vi "L42.vi"() -> ()   [LabVIEW 2014]
panel:
  in  "L42":dbl
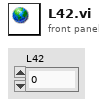
[diagram p1: front panel]
diagram:
